vi "Draw Legend.vi"(9 "State Data":T2, 10 "Properties:Draw Area Size":T1, 11 "Margin":i16) -> (0 "mask":u8[](array[numeric]), 1 "24-bit pixmap":u32[][](array[numeric]), 2 "Draw Position":cluster{"x":i16, "y":i16}, 3 "Legend Width":u32)   [LabVIEW 2018, in "PieChart.lvclass"]
uses:
  PieChart.lvclass
  <vilib>/Utility/miscctls.llb/LVFontTypeDef.ctl
  State Data.ctl
  <vilib>/Utility/miscctls.llb/LVBoundsTypeDef.ctl
  Pie info for Click.ctl
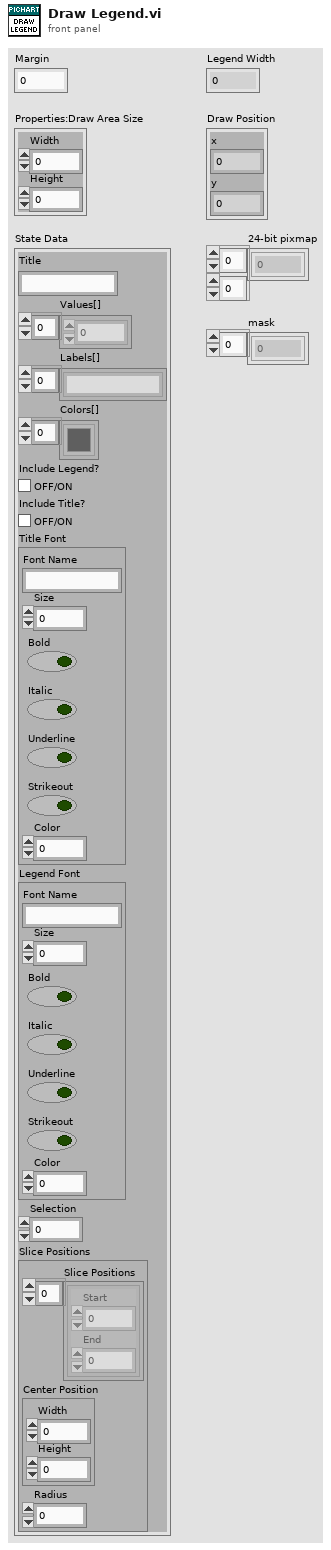
[diagram p1: front panel]
types:
  T1 = typedef "LVBoundsTypeDef.ctl" = cluster{"Width":u32, "Height":u32}
  T2 = typedef "PieChart.lvclass/State Data.ctl" = cluster{"Title":string, "Values[]":dbl[], "Labels[]":string[], "Colors[]":u32[], "Include Legend?":bool, "Include Title?":bool, "Title Font":T3, "Legend Font":T3, "Selection":i32, "Slice Positions":T4}
  T3 = typedef "LVFontTypeDef.ctl" = cluster{"Font Name":string, "Size":u16, "Bold":bool, "Italic":bool, "Underline":bool, "Strikeout":bool, "Color":u32}
  T4 = typedef "PieChart.lvclass/Pie info for Click.ctl" = cluster{"Slice Positions":cluster{"Start":i16, "End":i16}[], "Center Position":T1, "Radius":i16}
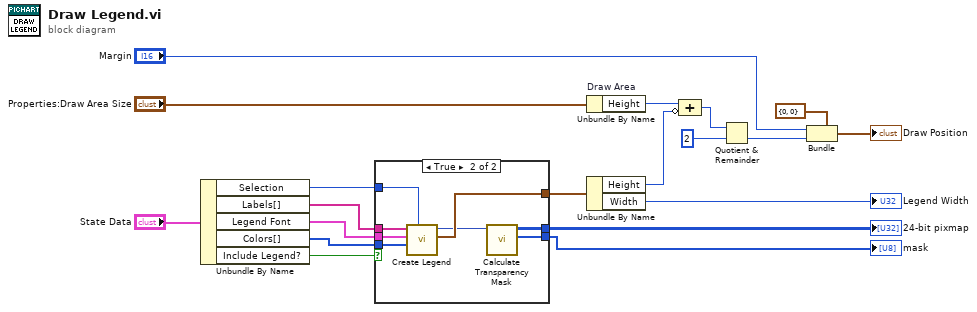
[diagram p0: block diagram]
diagram:
  n1 = Unbundle By Name("State Data") -> ("Selection"=w1:i32, "Labels[]"=w15:string[], "Legend Font"=w16:T3, "Colors[]"=w18:u32[], "Include Legend?"=w17:bool)
  n2 = case shown="True" w17 {
    tunnel: w16 -> [_ w27]
    tunnel: w15 -> [_ w26]
    tunnel: [_ w25] -> w8
    tunnel: [_ w22] -> w3
    tunnel: w18 -> [_ w24]
    tunnel: [_ w21] -> w10
    tunnel: w1 -> [_ w20]
    frame False {
    }
    frame True {
      n3 = call "Create Legend.vi"("Selection"=w20, "Colors[] (Use Default)"=w24, "Font"=w27, "Labels[]"=w26) -> ("Legend Box Size"=w25:cluster{"Width":u32, "Height":u32}, "Legend out"=w23:picture)  [unwired: 6 in]
      n4 = call "Calculate Transparency Mask.vi"("Picture in"=w23) -> ("mask"=w21:u8[], "24-bit pixmap"=w22:u32[][])  [unwired: 8 in, 1 out]
    }
  }
  "mask" <- w10
  "24-bit pixmap" <- w3
  n5 = Unbundle By Name "Draw Area"("Properties:Draw Area Size") -> ("Height"=w13:u32)
  n6 = Unbundle By Name(w8) -> ("Height"=w2:u32, "Width"=→"Legend Width":u32)
  n7 = Compound Arithmetic op=ADD(w13, invert w2) -> (w6:u32)
  n8 = Quotient & Remainder(x=w6, y=u32 2) -> (floor(x/y)=w9:u32)  [unwired: 1 out]
  n9 = Bundle(cluster=cluster{"x":i16, "y":i16} {"x"=0, "y"=0} ("top left point(0, 0)"), "x"="Margin", "y"=w9) -> (→"Draw Position":cluster{"x":i16, "y":i16})
